vi "WriteHSpeed.vi"(8 "error in":errorcluster, 9 "Reply length":i32=-1, 10 "write buffer":string, 11 "Python":T1) -> (0 "error out":errorcluster, 2 "read buffer":string, 3 "Python":T1)   [LabVIEW 2020]
uses:
  PythonCtrl.ctl
  Processors.ctl
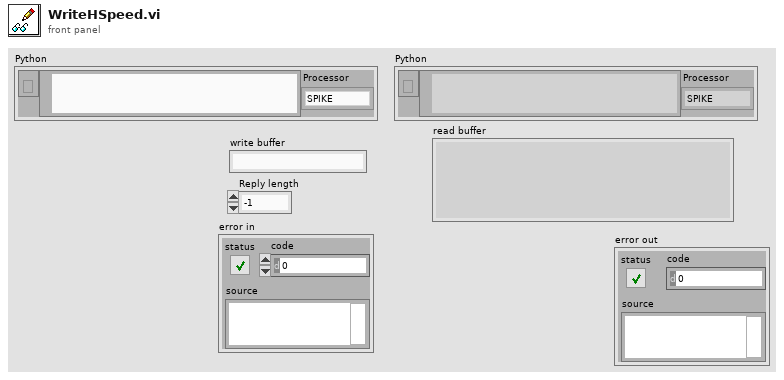
[diagram p1: front panel]
types:
  T1 = typedef "PythonCtrl.ctl" = cluster{"session":refnum<k35>, "PyPath":path, "Processor":T2}
  T2 = typedef "Processors.ctl" = enum16{"SPIKE", "Pi", "Pi_ssh", "OpenMV"}
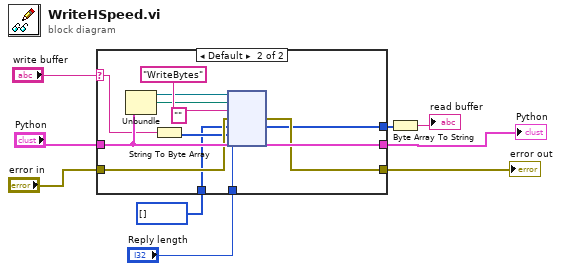
[diagram p0: block diagram]
diagram:
  n1 = case shown="Default" "write buffer" {
    selector: "write buffer" -> [_ w16]
    tunnel: "Python" -> [w11 w21]
    tunnel: "error in" -> [w10 w18]
    tunnel: [w11 w21] -> w5
    tunnel: [w10 w17] -> w4
    tunnel: "Reply length" -> [_ w15]
    tunnel: [_ w14] -> w2
    tunnel: u8[] [] ("unsigned byte array") -> [_ w12]
    frame "" {
    }
    frame Default {
      (unwired) "" ("function name")
      n2 = Unbundle(w21) -> ("session"=w20:refnum<k35>, "PyPath"=w19:path)  [unwired: 1 out]
      n3 = String To Byte Array(string=w16) -> (unsigned byte array=w13:u8[])
      n4 = node(w20, w19, "WriteBytes" ("function name"), w18, w12, w13, w15) -> (w17:errorcluster, w14:u8[])  [unwired: 2 in, 3 out]
    }
  }
  "Python" <- w5
  "error out" <- w4
  n5 = Byte Array To String(unsigned byte array=w2) -> (string=→"read buffer":string)
